vi "ApplyLayoutToObject.vi"(5 "scaling settings":T1={"scaling factor"={"horizontal"=1.0, "vertical"=1.0}, "scaling to ignore"=variant} {"scaling factor"."vertical" min=0.0; "scaling factor"."horizontal" min=0.0}, 7 "properties to ignore":variant, 8 "error in (no error)":errorcluster, 10 "GObj Refnum":refnum<vi>, 11 "Tab Control Layout in":refnum<class "Tab Control Layout.lvclass">) -> (0 "error out":errorcluster, 3 "Tab Control Layout out":refnum<class "Tab Control Layout.lvclass">)   [LabVIEW 2010, in "NI_SE_Front Panel Layout.lvlib" / "Tab Control Layout.lvclass"]
doc: "Apply layout information to the GObj Refnum."
uses:
  Tab Control Layout.lvclass
  Control Layout/Control Layout.lvclass
  Properties To Ignore.vi
  NI_SE_Front Panel Layout.lvlib
  XY Scaling Factor.ctl
  Scaling Factor_Options.ctl
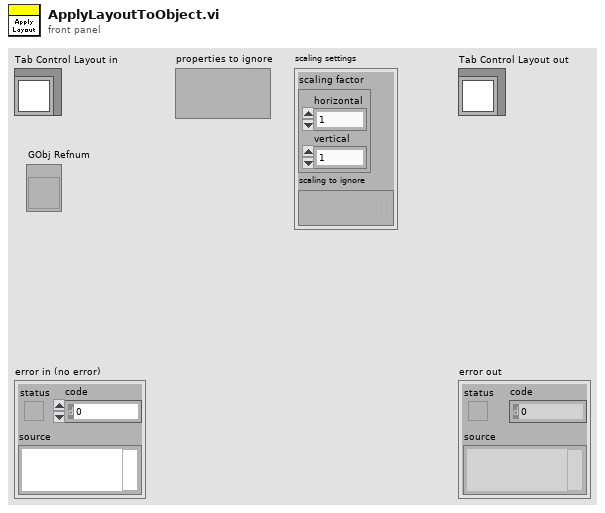
[diagram p1: front panel]
types:
  T1 = typedef "NI_SE_Front Panel Layout.lvlib/Scaling Factor_Options.ctl" = cluster{"scaling factor":T2, "scaling to ignore":variant}
  T2 = typedef "NI_SE_Front Panel Layout.lvlib/XY Scaling Factor.ctl" = cluster{"horizontal":dbl, "vertical":dbl}
  T3 = typedef "LVBoundsTypeDef.ctl" = cluster{"Width":u32, "Height":u32}
  T4 = enum32{"Size Tabs To Contents", "Size All Tabs to Largest Tab", "Fixed Tab Size"}
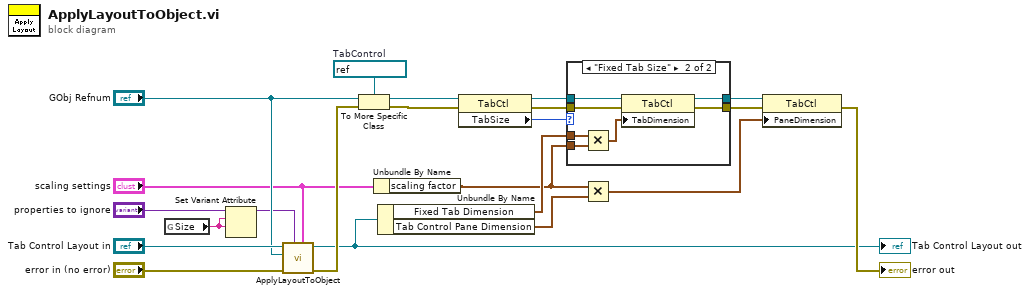
[diagram p0: block diagram]
diagram:
  w13 = refnum<vi> refnum  # TabControl
  n1 = global read "Properties To Ignore.vi" "Size"() -> (w1:string)
  n2 = Set Variant Attribute(Variant="properties to ignore", name=w1, value=w1) -> (Variant out=w14:variant)  [unwired: 1 in, 2 out]
  n3 = call-parent "ApplyLayoutToObject.vi"("scaling settings"="scaling settings", "properties to ignore"=w14, "error in (no error)"="error in (no error)", "GObj Refnum"="GObj Refnum", "Control Layout in"="Tab Control Layout in") -> ("error out"=w20:errorcluster, "Control Layout out"=w18:refnum<class "Tab Control Layout.lvclass">)  [unwired: 5 in]
  "Tab Control Layout out" <- w18
  n4 = To More Specific Class(target class=w13, reference="GObj Refnum", error in=w20) -> (specific class reference=w12:refnum<vi>, error out=w11:errorcluster)
  n5 = Unbundle By Name("scaling settings") -> ("scaling factor"=w2:T2)
  n6 = Unbundle By Name(w18) -> ("Fixed Tab Dimension"=w7:T3, "Tab Control Pane Dimension"=w4:T3)
  n7 = property class="TabCtl"(reference=w12, error in=w11) -> (reference out=w8:refnum<vi>, error out=w9:errorcluster, "TabSize"=w10:T4)
  n8 = case shown="\"Fixed Tab Size\"" w10 {
    tunnel: w9 -> [w23 w30]
    tunnel: w8 -> [w24 w31]
    tunnel: [w24 w28] -> w6
    tunnel: [w23 w29] -> w5
    tunnel: w7 -> [_ w26]
    tunnel: w2 -> [_ w27]
    frame Default {
    }
    frame "Fixed Tab Size" {
      n9 = Multiply(x=w26, y=w27) -> (x*y=w25:T2)
      n10 = property class="TabCtl"(reference=w31, error in=w30, "TabDimension"=w25) -> (reference out=w28:refnum<vi>, error out=w29:errorcluster)
    }
  }
  n11 = Multiply(x=w2, y=w4) -> (x*y=w3:T2)
  n12 = property class="TabCtl"(reference=w6, error in=w5, "PaneDimension"=w3) -> (error out=→"error out":errorcluster)  [unwired: 1 out]
